vi "Pfeiffer Vacuum Integrated Sensors Read Data.vi"(8 "error in (no error)":errorcluster, 9 "PV Integrated pressure Sensor - Cluster":T1={"Parameter"=enum." Pressure 1 value [hPa] (740) (default)", "Parameter\nread only<->describe"=FALSE, "Correction facktor\n(0,20 - 9,90) "=1.0, "Pressure set point (hPa)\n0 => ur (p<1,0e-5 hPa)\n850 - 1250 hPa"=0, "Pressure switch\npoint (hPa)"=1.0, "Pressure HV enable (IKT010 only)"=0} {"Pressure HV enable (IKT010 only)" items=["off", "on", "on above TMP speed switchpoint", "on below pressure 2 switchpoint"]; "Pressure switch\npoint (hPa)" min=5e-10 max=2000.0 step=1.0 format="%_3e"; "Pressure set point (hPa)\n0 => ur (p<1,0e-5 hPa)\n850 - 1250 hPa" min=0 max=2050 step=1; "Correction facktor\n(0,20 - 9,90)" min=0.2 max=9.9 step=0.01 format="%.2f"}, 10 "Adress of unit":u16=1 min=1 max=999 step=1, 11 "VISA session in":refnum<visa-resource-name>) -> (0 "error out":errorcluster, 3 "response (data)":string)   [LabVIEW 2021]
doc: "This VI is an example of how to use the Pfeiffer Vacuum subVIs programmatically. This VI first initializes the instrument, takes measurements, then closes the instrument."
uses:
  <instrlib>/Pfeiffer Vacuum/Public/Turbopumps/PV Integrated Pressure Sensors - Cluster.ctl
  <instrlib>/Pfeiffer Vacuum/Pfeiffer Vacuum.lvlib
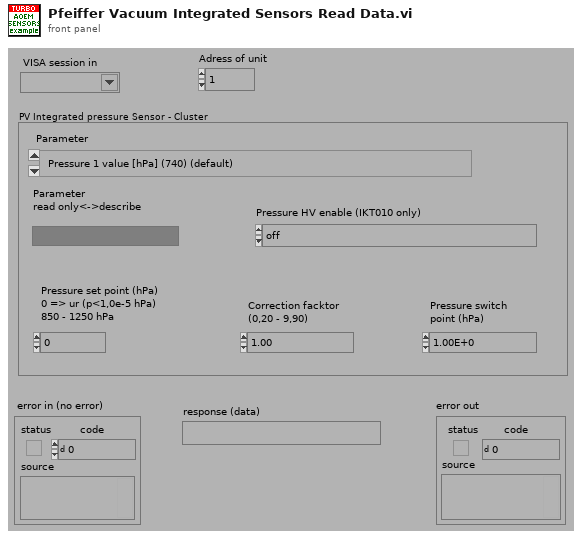
[diagram p1: front panel]
types:
  T1 = typedef "Pfeiffer Vacuum.lvlib/PV Integrated Pressure Sensors - Cluster.ctl" = cluster{"Parameter":enum16{" Pressure 1 switchpoint [hPa] (730) (default)", " Pressure 2 switchpoint [hPa] (732)", " Name of sensor 1 (739)", " Pressure 1 value [hPa] (740) (default)", " Correction factor 1 (742)", " Name of sensor 2 (749)", " Pressure 2 value [hPa] (750)", " Correction factor 2 (752)", " Pressure HV enable (IKT010 only) (041)"}, "Parameter\nread only<->describe":bool, "Correction facktor\n(0,20 - 9,90) ":sgl, "Pressure set point (hPa)\n0 => ur (p<1,0e-5 hPa)\n850 - 1250 hPa":i16, "Pressure switch\npoint (hPa)":dbl, "Pressure HV enable (IKT010 only)":u16}
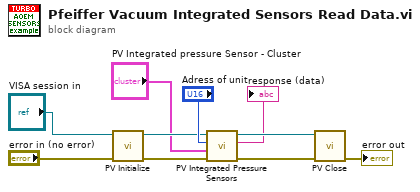
[diagram p0: block diagram]
diagram:
  n1 = call <instrlib>:"PV Initialize.vi"("error in (no error)"="error in (no error)", "VISA session in"="VISA session in") -> ("error out"=w4:errorcluster, "VISA session out"=w3:refnum<visa-resource-name>)  [unwired: 8 in]
  n2 = call <instrlib>:"PV Integrated Pressure Sensors.vi"("error in (no error)"=w4, "PV Integrated pressure Sensor - Cluster"="PV Integrated pressure Sensor - Cluster", "Adress of unit"="Adress of unit", "VISA session"=w3) -> ("error out"=w10:errorcluster, "response (data)"=→"response (data)":string, "dup VISA session"=w9:refnum<visa-resource-name>)  [unwired: 5 in]
  n3 = call <instrlib>:"PV Close.vi"("VISA session"=w9, "error in (no error)"=w10) -> ("error out"=→"error out":errorcluster)  [unwired: 13 in]
